vi "ConvertMatlabDataValueToArray.vi"(10 "Original Value":variant, 11 "Data":variant) -> (3 "Array":variant)   [LabVIEW 2017]
uses:
  Types/MatlabDataTypeDescriptorEnum.ctl
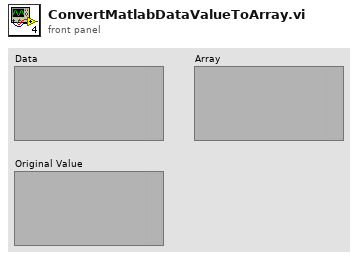
[diagram p1: front panel]
types:
  T1 = typedef "MatlabDataType.ctl" = enum16{"NotAMatlabType", "Real", "Complex", "String", "Boolean"}
  T2 = typedef "MatlabDataTypeDescriptorEnum.ctl" = enum16{"Not a collection", "Array", "Waveform"}
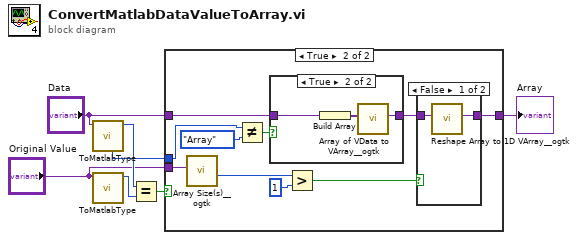
[diagram p0: block diagram]
diagram:
  n1 = call "ToMatlabType.vi"("Value"="Data") -> ("MatlabType"=w6:T1, "DataType Collection"=w1:T2)  [unwired: 6 in, 3 out]
  n2 = call "ToMatlabType.vi"("Value"="Original Value") -> ("MatlabType"=w7:T1)  [unwired: 6 in, 4 out]
  n3 = Equal?(x=w6, y=w7) -> (x = y?=w3:bool)
  n4 = case shown="True" w3 {
    tunnel: "Original Value" -> [w8 w18]
    tunnel: "Data" -> [_ w11]
    tunnel: [w8 w14] -> w2
    tunnel: w1 -> [_ w9]
    frame False {
    }
    frame True {
      n5 = call <userlib>:"Array Size(s)__ogtk.vi"("Array"=w18) -> ("N dims"=w15:u32)  [unwired: 8 in, 2 out]
      n6 = Not Equal?(x=w9, y=MatlabDataTypeDescriptorEnum."Array") -> (x != y?=w12:bool)
      n7 = case shown="True" w12 {
        tunnel: w11 -> [w19 w22]
        tunnel: [w19 w20] -> w10
        frame False {
        }
        frame True {
          n8 = Build Array(w22) -> (w21:variant[])
          n9 = call <userlib>:"Array of VData to VArray__ogtk.vi"("1D Array of VData"=w21) -> ("VArray"=w20:variant)  [unwired: 9 in, 1 out]
        }
      }
      n10 = Greater?(x=w15, y=u32 1) -> (0:w17:bool)
      n11 = case shown="False" w17 {
        tunnel: w10 -> [w24 w25]
        tunnel: [w23 w25] -> w14
        frame False {
          n12 = call <userlib>:"Reshape Array to 1D VArray__ogtk.vi"("MultiD Array"=w24) -> ("1D VArray"=w23:variant)  [unwired: 8 in, 2 out]
        }
        frame True {
        }
      }
    }
  }
  "Array" <- w2
